vi "FT_Get_Device_Info_Detail.vi"(0 "Device Index":u32) -> (1 "FT_Status":u32(ring) items=["FT_OK", "FT_INVALID_HANDLE", "FT_DEVICE_NOT_FOUND", "FT_DEVICE_NOT_OPENED", "FT_IO_ERROR", "FT_INSUFFICIENT_RESOURCES", "FT_INVALID_PARAMETER", "FT_INVALID_BAUD_RATE", "FT_DEVICE_NOT_OPENED_FOR_ERASE", "FT_DEVICE_NOT_OPENED_FOR_WRITE", "FT_FAILED_TO_WRITE_DEVICE", "FT_EEPROM_READ_FAILED", "FT_EEPROM_WRITE_FAILED", "FT_EEPROM_ERASE_FAILED", "FT_EEPROM_NOT_PRESENT", "FT_EEPROM_NOT_PROGRAMMED", "FT_INVALID_ARGS", "FT_NOT_SUPPORTED", "FT_OTHER_ERROR"], 2 "Device Info Node":T1 {"FT_Handle" format="%.0x"; "LocID" format="%.0x"; "PID" format="%.0x"; "VID" format="%.0x"; "Type" items=["FT232B-FT245B", "FT8U232AM-FT8U245AM", "FT8U100AX", "UNKNOWN", "FT2232", "FT232R", "FT2232H", "FT4232H", "FT232H"]})   [LabVIEW 2019, in "D2XX.lvlib"]
uses:
  D2XX.lvlib
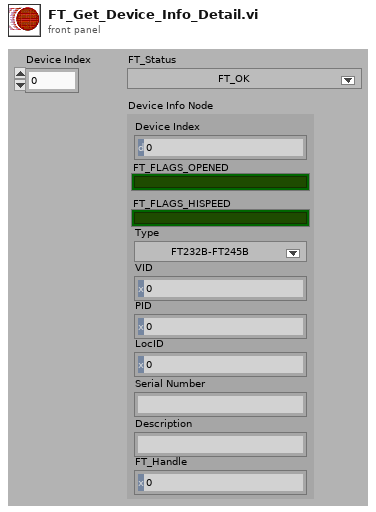
[diagram p1: front panel]
types:
  T1 = cluster{"Device Index":u32, "FT_FLAGS_OPENED":bool, "FT_FLAGS_HISPEED":bool, "Type":u32, "VID":u32, "PID":u32, "LocID":i32, "Serial Number":string, "Description":string, "FT_Handle":u32}
  T2 = cluster{"Device Index":u32, bool, bool, "Type":u32, u32, u32, "LocID":i32, "Serial Number":string, "Description":string, "FT_Handle":u32}
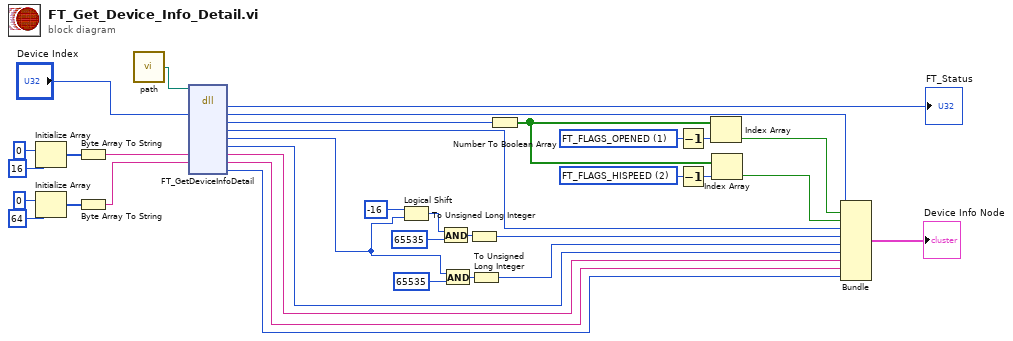
[diagram p0: block diagram]
diagram:
  w2 = u32 2 items=["FT_FLAGS_OPENED"=1, "FT_FLAGS_HISPEED"=2] ("Flags")
  w5 = u32 1 items=["FT_FLAGS_OPENED"=1, "FT_FLAGS_HISPEED"=2] ("Flags")
  n1 = Initialize Array(u8 0, 16 ("dimension size")) -> (w28:u8[])
  n2 = Initialize Array(u8 0, 64 ("dimension size")) -> (w26:u8[])
  n3 = Byte Array To String(unsigned byte array=w28) -> (string=w25:string)
  n4 = Byte Array To String(unsigned byte array=w26) -> (string=w24:string)
  n5 = call "path.vi"() -> ("lib path"=w1:path)
  n6 = dll-call lib="FTD2XX.dll" fn="FT_GetDeviceInfoDetail"(path in=w1, "Device Index"="Device Index", "Serial Number"=w25, "Description"=w24) -> ("FT_Status"=→"FT_Status":u32, "Device Index"=w33:u32, "Flags"=w10:u32, "Type"=w32:u32, "Device ID"=w11:u32, "LocID"=w12:i32, "Serial Number"=w31:string, "Description"=w13:string, "FT_Handle"=w30:u32)  [unwired: 7 in, 2 out]
  n7 = Logical Shift(y=-16, x=w11) -> (x << y=w19:u32)
  n8 = And(x=w19, y=u32 65535) -> (x .and. y?=w17:u32)
  n9 = And(x=w11, y=u32 65535) -> (x .and. y?=w15:u32)
  n10 = To Unsigned Long Integer(number=w17) -> (unsigned 32bit integer=w16:u32)
  n11 = To Unsigned Long Integer(number=w15) -> (unsigned 32bit integer=w14:u32)
  n12 = Number To Boolean Array(number=w10) -> (Boolean array=w8:bool[])
  n13 = Decrement(x=w5) -> (x-1=w4:u32)
  n14 = Decrement(x=w2) -> (x-1=w3:u32)
  n15 = Index Array(array=w8, index=w4) -> (element=w9:bool)
  n16 = Index Array(array=w8, index=w3) -> (element=w7:bool)
  n17 = Bundle("Device Index"=w33, w9, w7, "Type"=w32, w16, w14, "LocID"=w12, "Serial Number"=w31, "Description"=w13, "FT_Handle"=w30) -> (→"Device Info Node":T2)  [unwired: 1 in]
